vi "Build.vi"(8 "error in (no error)":errorcluster, 10 "Transfer Group in":refnum<class "Transfer Group.lvclass">, 11 "Type Converter in":refnum<class "String Type Buffer Converter.lvclass">) -> (0 "error out":errorcluster, 2 "Transfer Group out":refnum<class "Transfer Group.lvclass">, 3 "Type Converter out":refnum<class "String Type Buffer Converter.lvclass">)   [LabVIEW 2017, in "String Type Buffer Converter.lvlib" / "String Type Buffer Converter.lvclass"]
uses:
  String Type Buffer Converter.lvclass
  Builds/Data Sharing Framework/Current/Data Sharing Framework Core/DSF Core.lvlibp/Engine/Classes/Transfer Group/Transfer Group.lvclass
  String Type Buffer Converter.lvclass/String Type Buffer Converter.ctl
  Builds/Data Sharing Framework/Current/Data Sharing Framework Core/DSF Core.lvlibp/Engine/Classes/Buffer/Read Buffer String.vi
  Builds/Data Sharing Framework/Current/Data Sharing Framework Core/DSF Core.lvlibp/Engine/Classes/Buffer/Write Buffer String.vi
  Builds/Data Sharing Framework/Current/Data Sharing Framework Core/DSF Core.lvlibp/Engine/Classes/Buffer/Buffer.lvclass
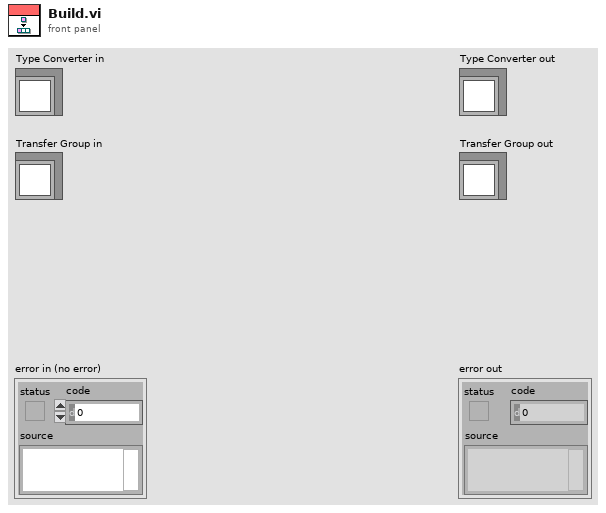
[diagram p1: front panel]
types:
  T1 = typedef "String Type Buffer Converter.lvlib/String Type Buffer Converter.lvclass/Conversion.ctl" = cluster{"conversion blocks":T2[]}
  T2 = typedef "String Type Buffer Converter.lvlib/String Type Buffer Converter.lvclass/Conversion Block.ctl" = cluster{"engine block descriptor":T3, "string block descriptor":T3, "engine byte order":enum16{"big-endian, network order", "native, host order", "little-endian"}, "string byte order":enum16{"big-endian, network order", "native, host order", "little-endian"}, "count":u64}
  T3 = typedef "DSF Core.lvlibp/Buffer.lvclass/Channel Descriptor.ctl" = cluster{"buffer offset":u64, "data type":T4}
  T4 = typedef "DSF Core.lvlibp/DSF Data Type.ctl" = enum8{"Bool", "SGL", "DBL", "I8", "I16", "I32", "I64", "U8", "U16", "U32", "U64"}
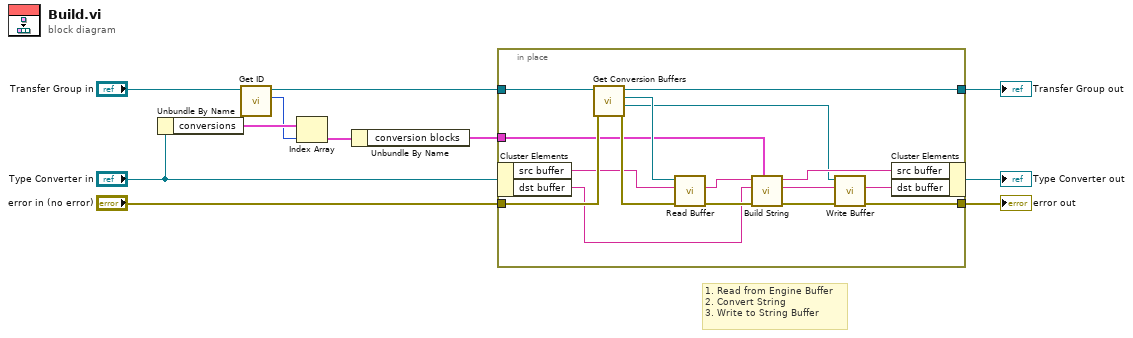
[diagram p0: block diagram]
diagram:
  # "1. Read from Engine Buffer\n2. Convert String\n3. Write to String Buffer"
  n1 = Unbundle By Name("Type Converter in") -> ("conversions"=w10:T1[])
  n2 = call "Get ID.vi"("Transfer Group in"="Transfer Group in") -> ("id"=w7:i32, "Transfer Group out"=w3:refnum<class "Transfer Group.lvclass">)  [unwired: 9 in]
  n3 = Index Array(array=w10, index=w7) -> (element=w9:T1)
  n4 = Unbundle By Name(w9) -> ("conversion blocks"=w8:T2[])
  n5 = in-place {
    in-place-border: w8 -> [w12]
    in-place-border: [w21] -> w5
    in-place-border: "error in (no error)" -> [w20]
    in-place-border: w3 -> [w19]
    in-place-border: [w14] -> w2
    n6 = in-place-cluster #1("Type Converter in") -> ("src buffer"=w16:string, "dst buffer"=w17:string)
    n7 = call "Get Conversion Buffers.vi"("error in (no error)"=w20, "Transfer Group in"=w19) -> ("error out"=w18:errorcluster, "string Buffer"=w13:refnum<class "Buffer.lvclass">, "engine Buffer"=w15:refnum<class "Buffer.lvclass">, "Transfer Group out"=w14:refnum<class "Transfer Group.lvclass">)  [unwired: 6 in]
    n8 = call-poly "Read Buffer.vi"("error in (no error)"=w18, "dst string in"=w16, "Buffer in"=w15) -> ("error out"=w23:errorcluster, "dst string out"=w27:string)  [unwired: 5 in, 2 out]
    n9 = call "Build String.vi"("conversion blocks"=w12, "error in (no error)"=w23, "dst buffer in"=w17, "src buffer in"=w27) -> ("error out"=w22:errorcluster, "dst buffer out"=w26:string, "src buffer out"=w24:string)  [unwired: 5 in]
    n10 = call-poly "Write Buffer.vi"("error in (no error)"=w22, "src string in"=w26, "Buffer in"=w13) -> ("error out"=w21:errorcluster, "src string out"=w25:string)  [unwired: 5 in, 2 out]
    n11 = in-place-cluster #1("src buffer"=w24, "dst buffer"=w25) -> (→"Type Converter out":refnum<class "String Type Buffer Converter.lvclass">)
  }
  "error out" <- w5
  "Transfer Group out" <- w2
